vi "禹山溶解氧校准.vi"() -> ()   [LabVIEW 2016, in "斯坦道多参数.lvlib"]
uses:
  <vilib>/Utility/miscctls.llb/LVPointTypeDef.ctl
  <vilib>/Analysis/NI_AALBase.lvlib
  <vilib>/Analysis/NI_AALPro.lvlib
  <vilib>/Utility/config.llb/NI_LVConfig.lvlib
panel:
  out "第二点信号值":dbl
  out "第一点信号值":dbl
  out "通讯状态":string
  in  "盐度自动获取":bool
  in  "大气压补偿":dbl format="%#.2f"
  in  "盐度补偿":dbl format="%#.2f"
  out "DO %":dbl caption="饱和度值" format="%#.2f"
  out "第二点校准值":dbl
  out "第一点校准值":dbl
  out "最小值":sgl format="%.2g"
  out "最大值":sgl format="%.2g"
  in  "校准停止":bool
  in  "校准模式":u16(ring) items=["两点校准", "单点校准"]
  in  "标液2":dbl
  in  "标液1":dbl
  out "波形图表":dbl(graph) caption="历史曲线"
  out "温度测量值":dbl caption="温度" format="%#.2f"
  out "变异系数":dbl format="%.6g"
  out "standard deviation":dbl caption="标准差" format="%0.2f"
  out "mean":dbl caption="均值" format="%0.2f"
  out "提示":string
  in  "校准启动":bool
  out "DO mg/L":dbl caption="测试值" format="%#.2f"
  out "电极斜率":dbl format="%#.6f"
  out "电极零点":dbl format="%#.6f"
  # "溶解氧电极设定"
  # "℃"
  # "%"
  # "mg/L"
  # "kPa"
  # "请选择校准模式:"
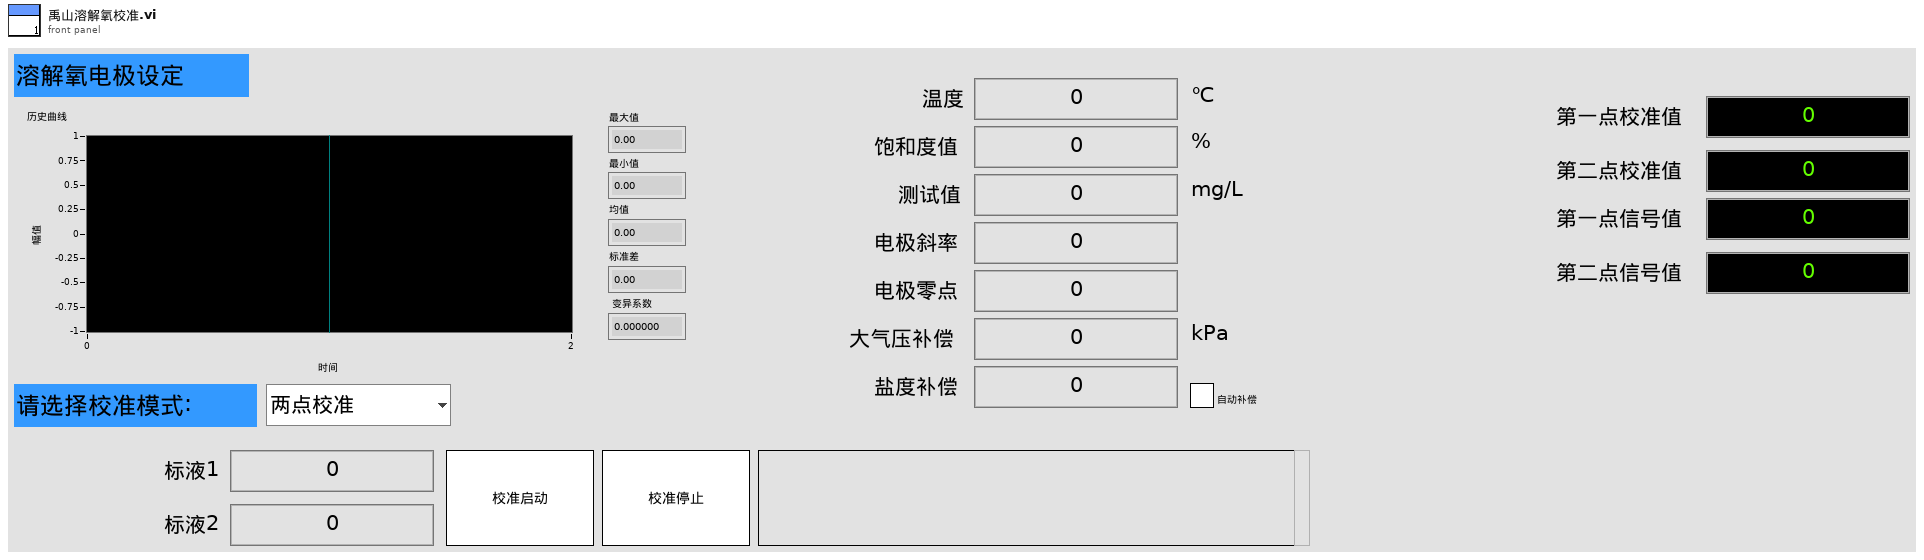
[diagram p1: front panel]
types:
  T1 = typedef "LVPointTypeDef.ctl" = cluster{"Horizontal":i16, "Vertical":i16}
  T2 = typedef "NI_LVConfig.lvlib/Config Data RefNum.ctl" = refnum<k1>
  T3 = enum8{"Enabled", "Disabled", "Disabled and Grayed Out"}
  T4 = cluster{"ph":bool, "DO":bool, "Cond":bool, "Turb":bool, "叶绿素a":bool, "藻密度":bool, "ORP":bool}
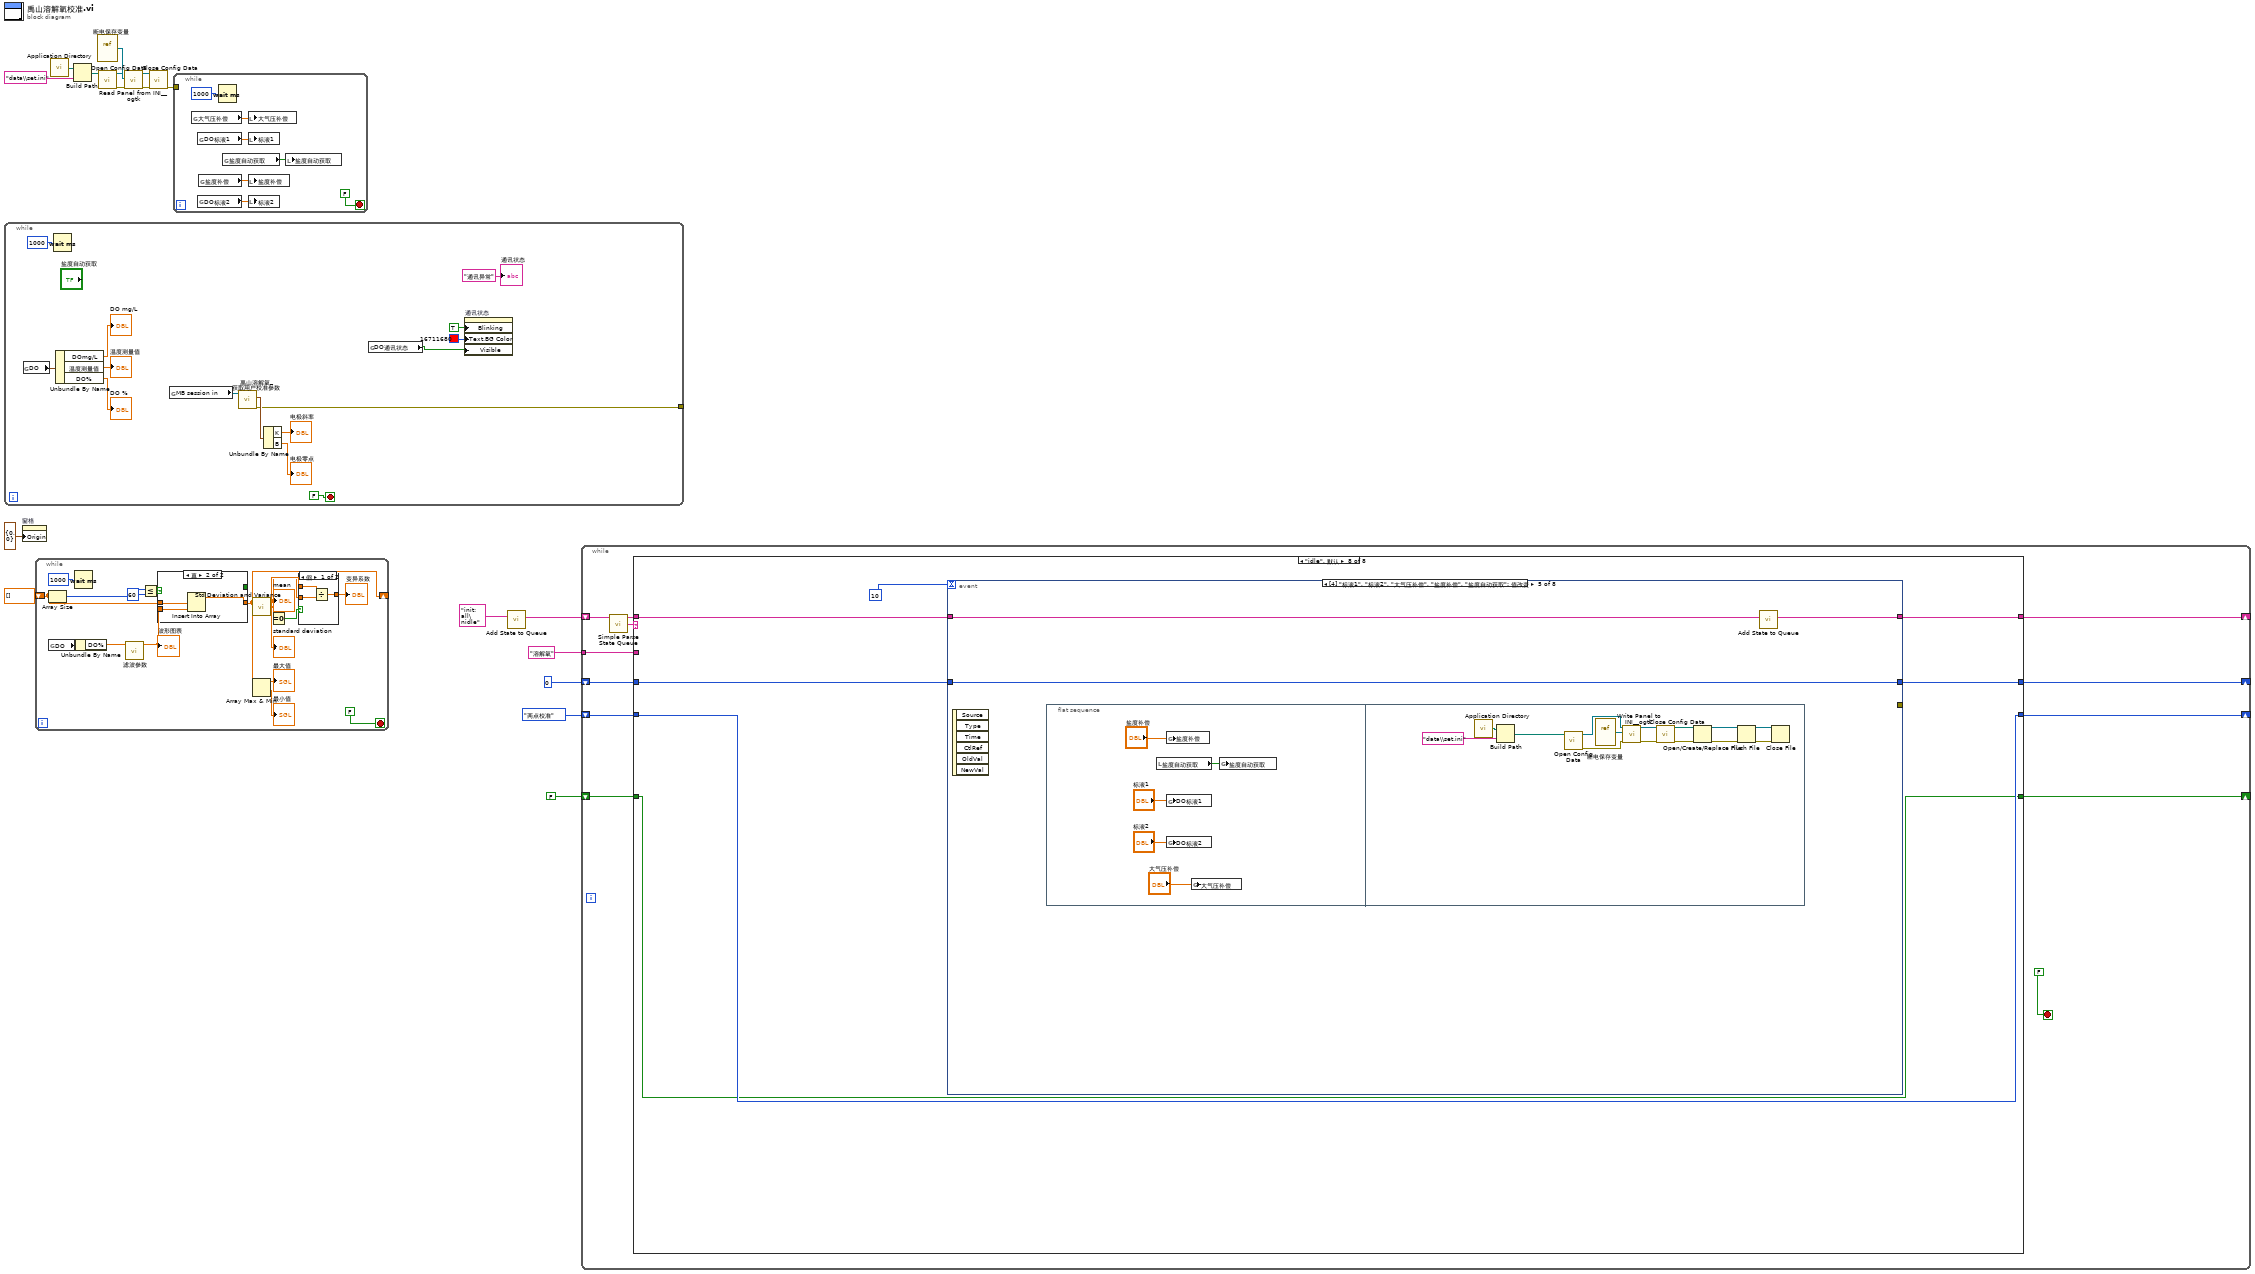
[diagram p0: block diagram]
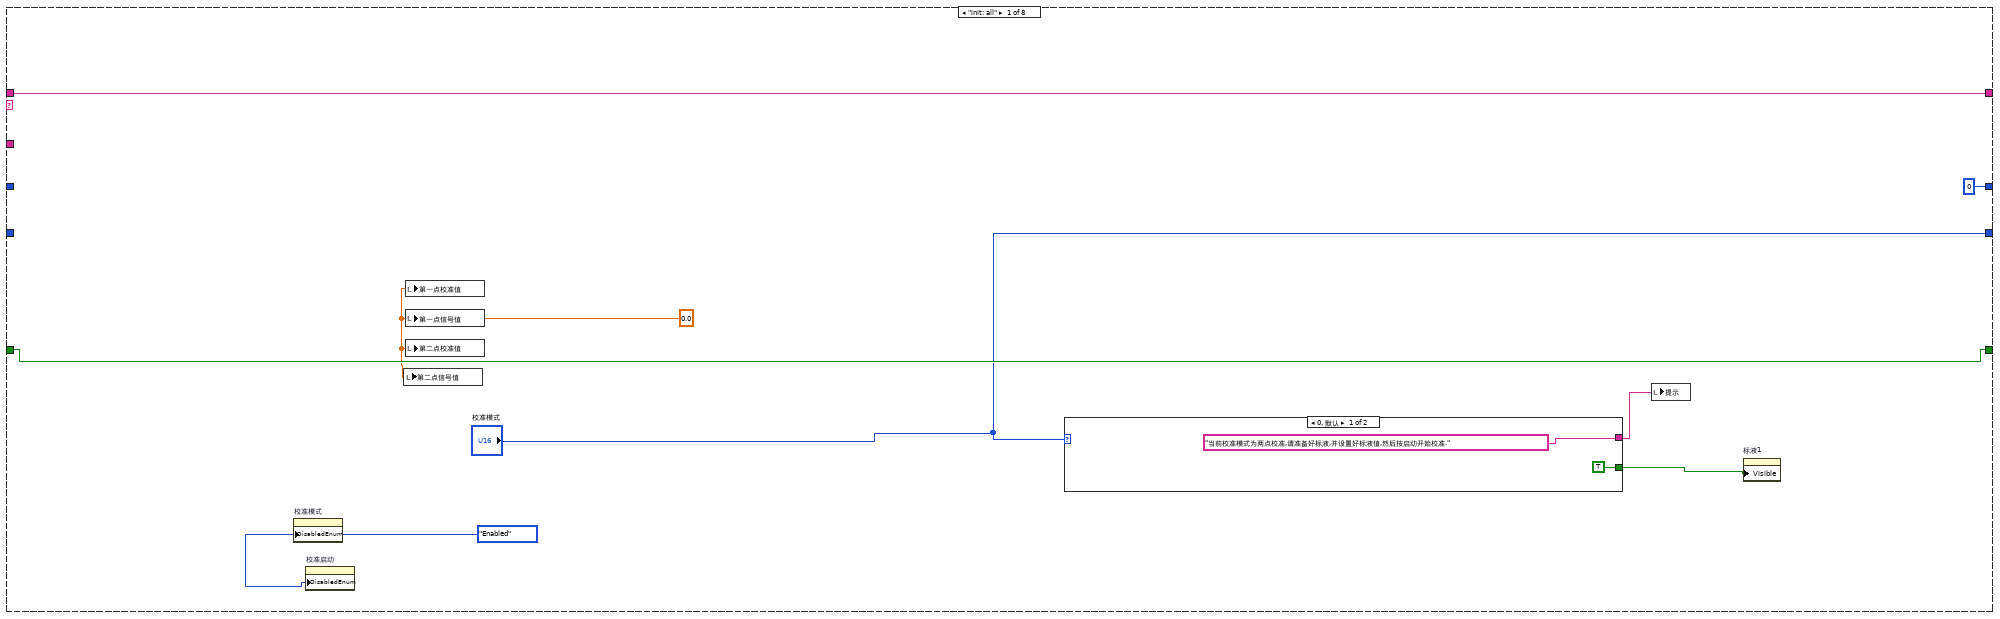
[diagram p2: hidden frame]
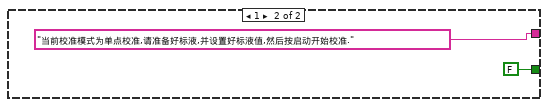
[diagram p3: hidden frame]
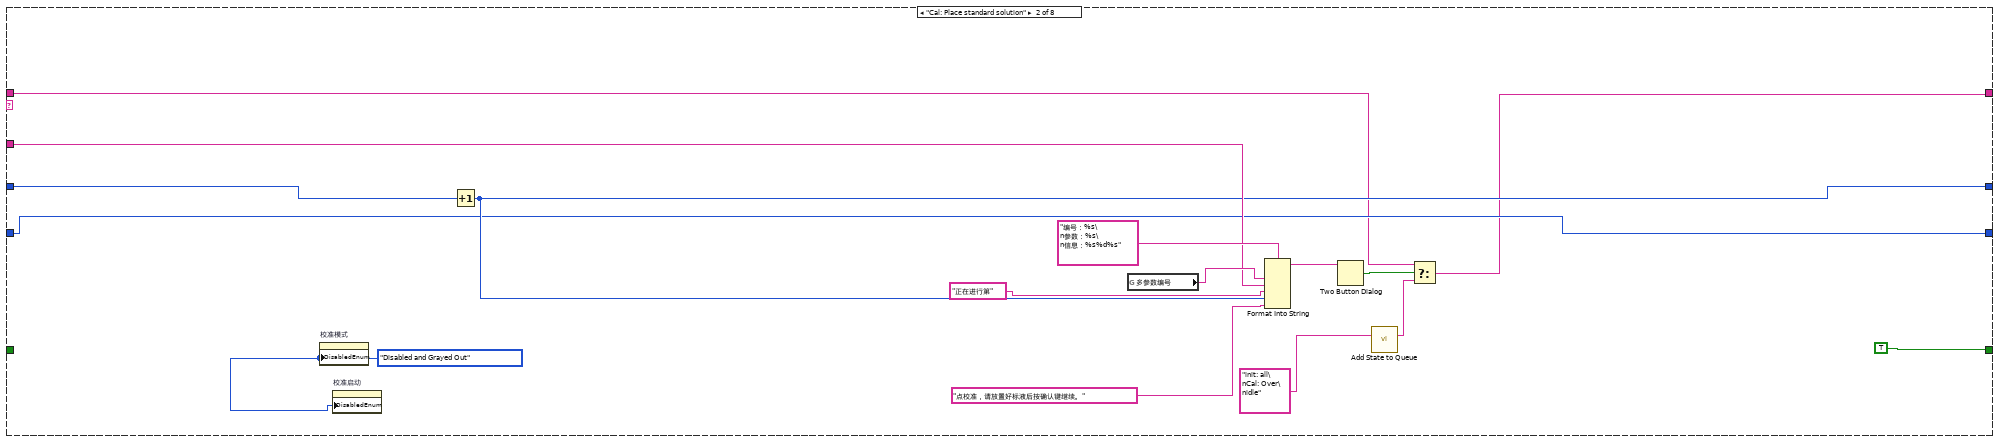
[diagram p4: hidden frame]
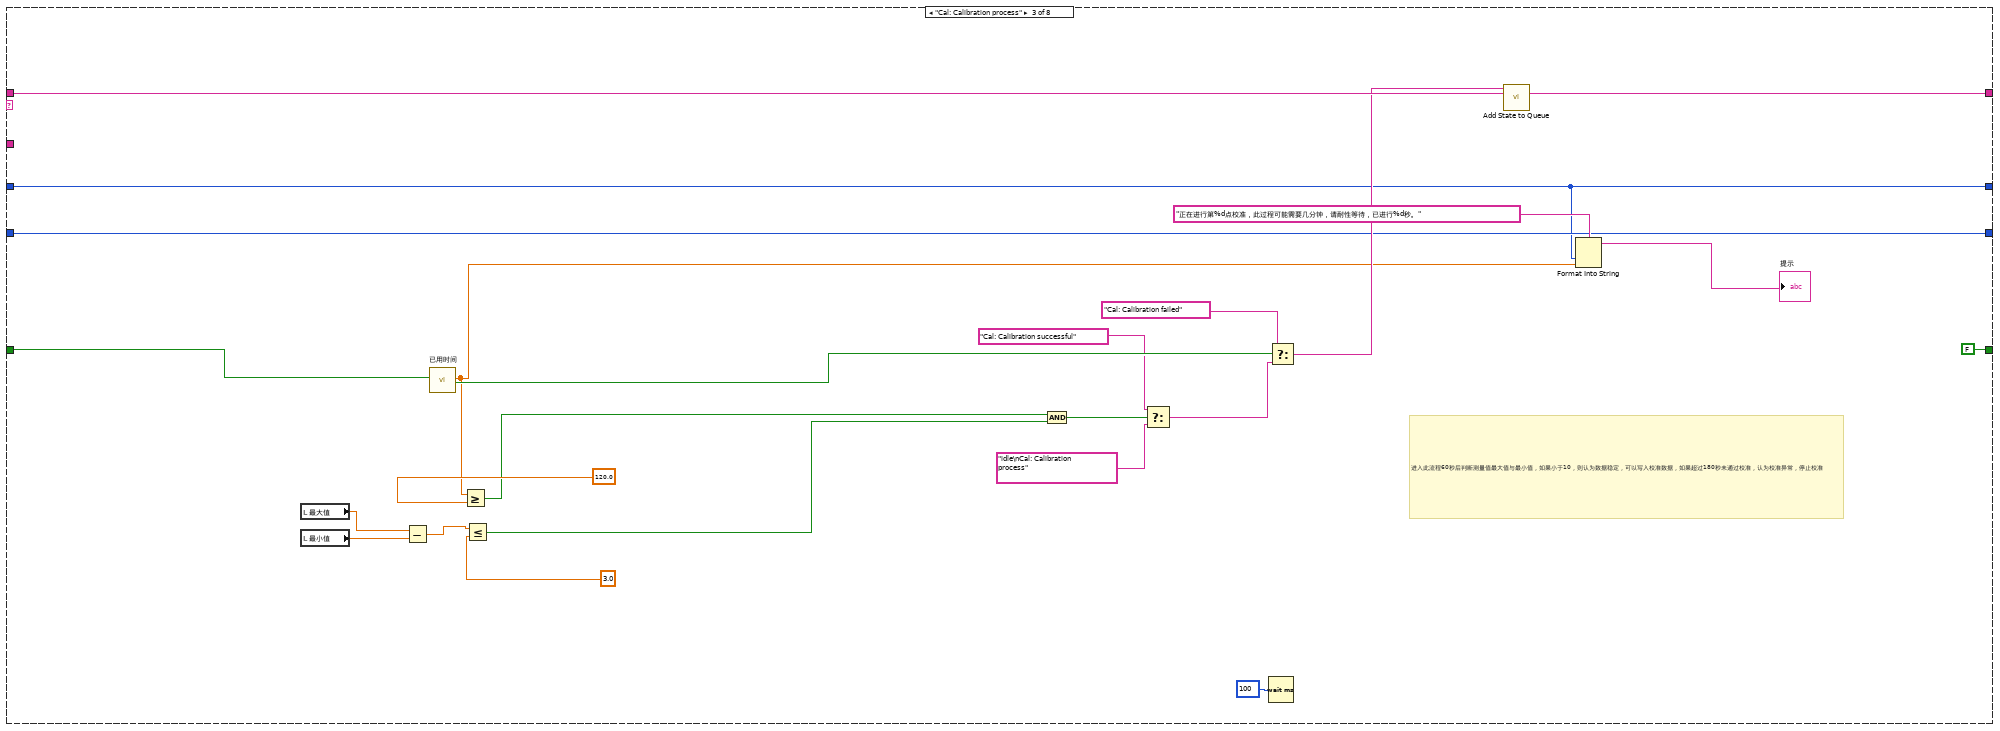
[diagram p5: hidden frame]
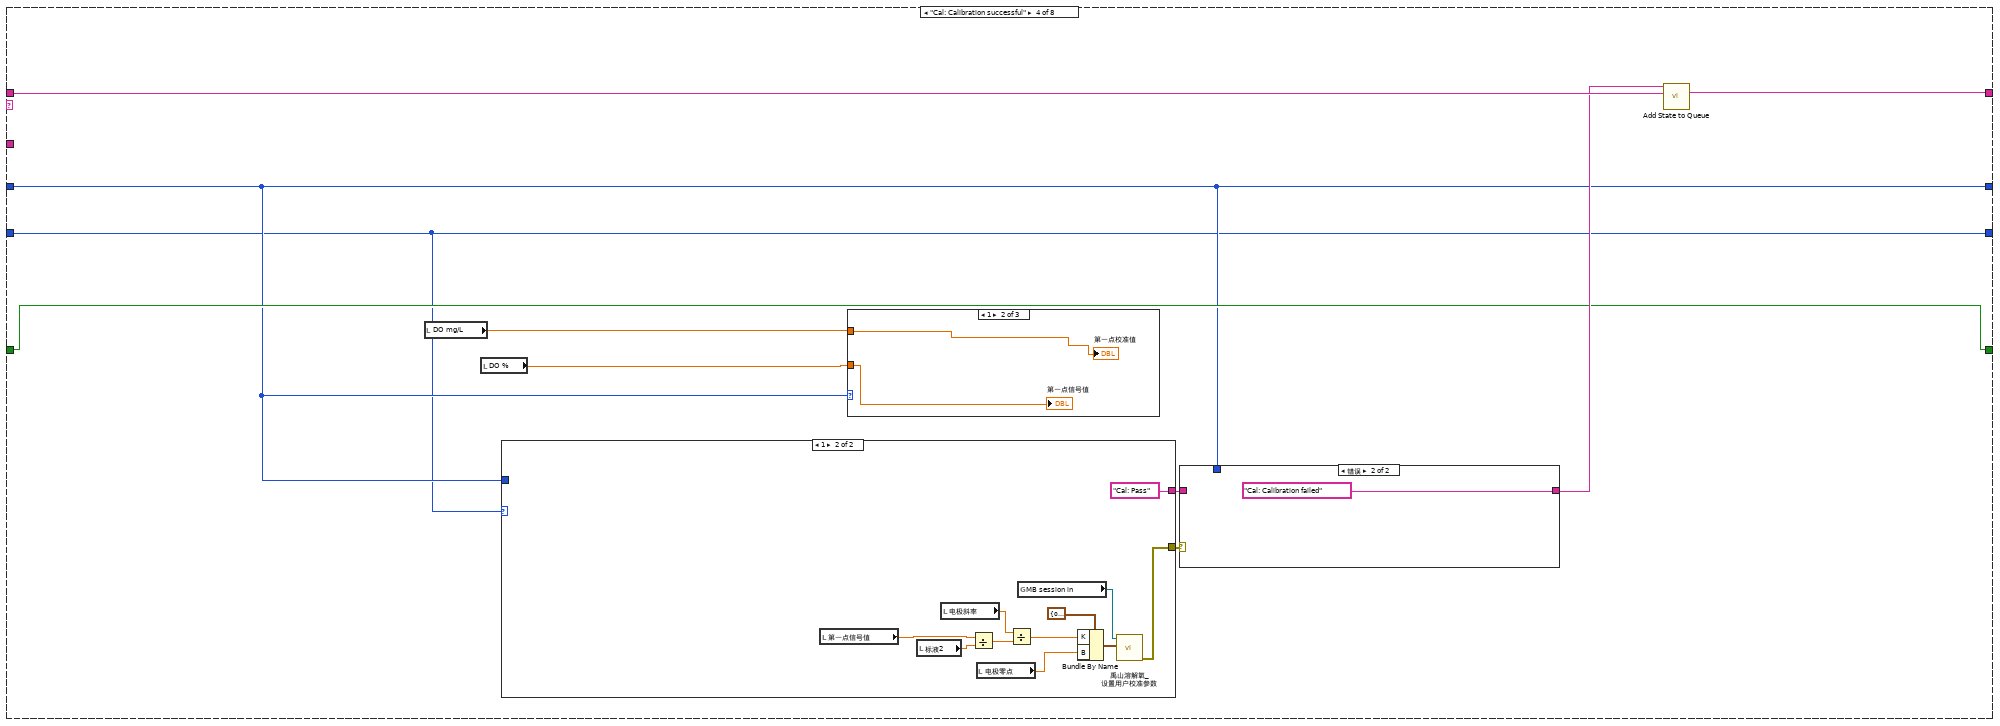
[diagram p6: hidden frame]
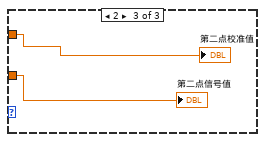
[diagram p8: hidden frame]
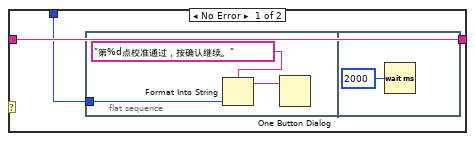
[diagram p9: hidden frame]
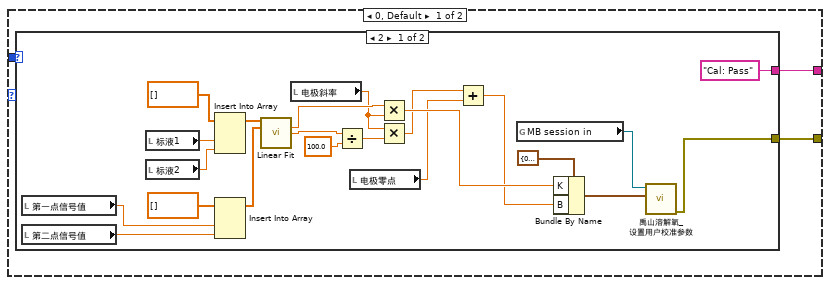
[diagram p10: hidden frame]
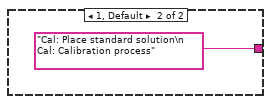
[diagram p11: hidden frame]
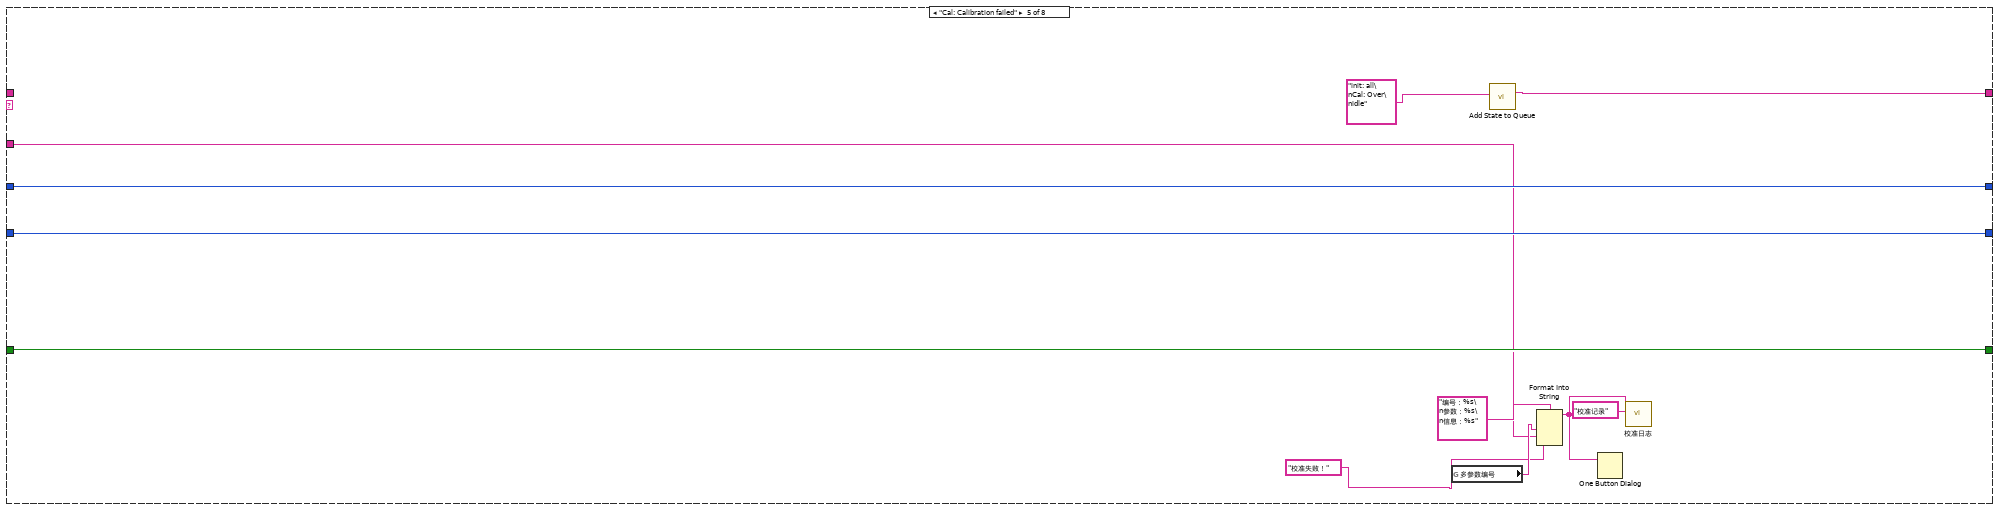
[diagram p12: hidden frame]
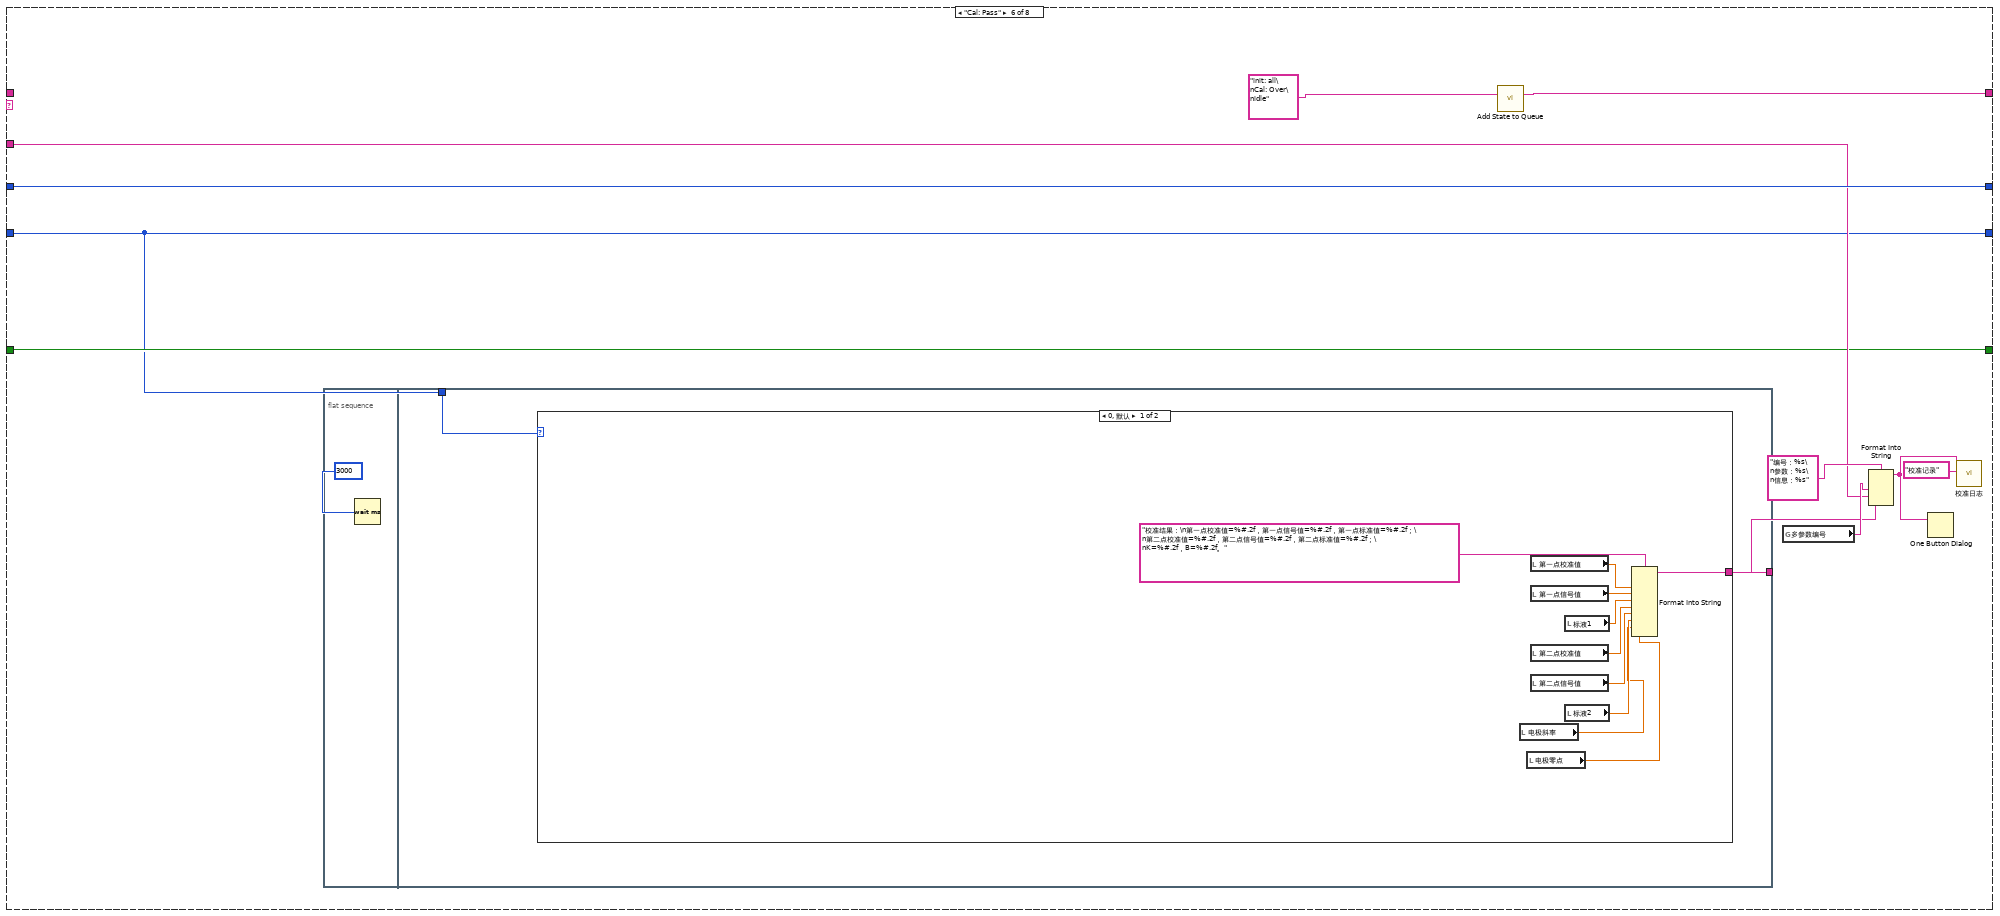
[diagram p13: hidden frame]
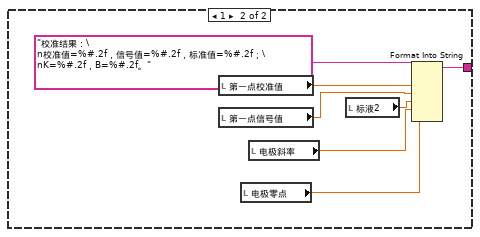
[diagram p14: hidden frame]
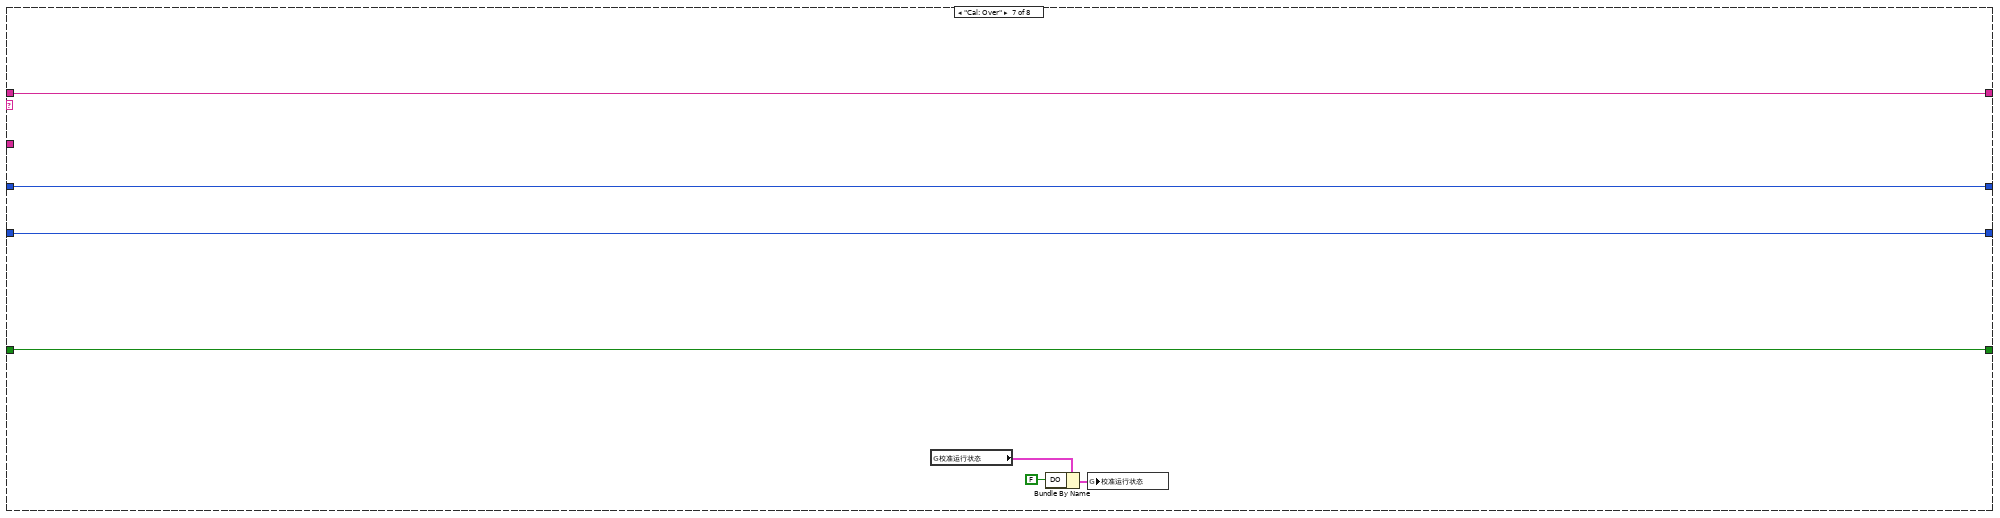
[diagram p15: hidden frame]
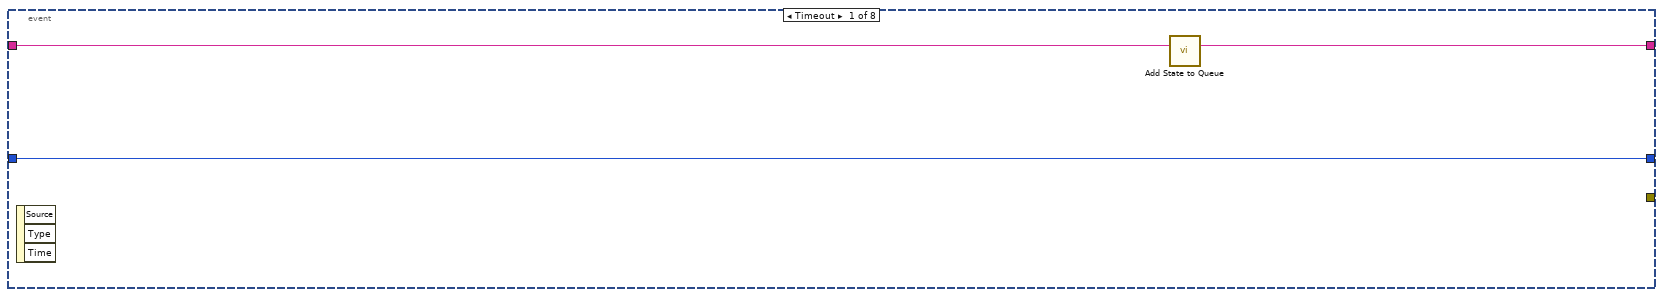
[diagram p16: hidden frame]
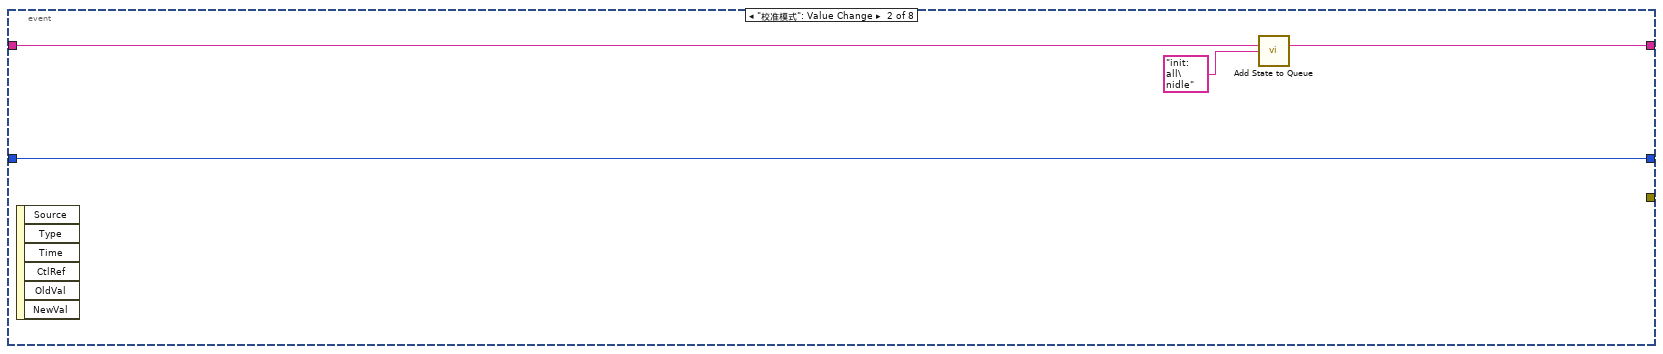
[diagram p17: hidden frame]
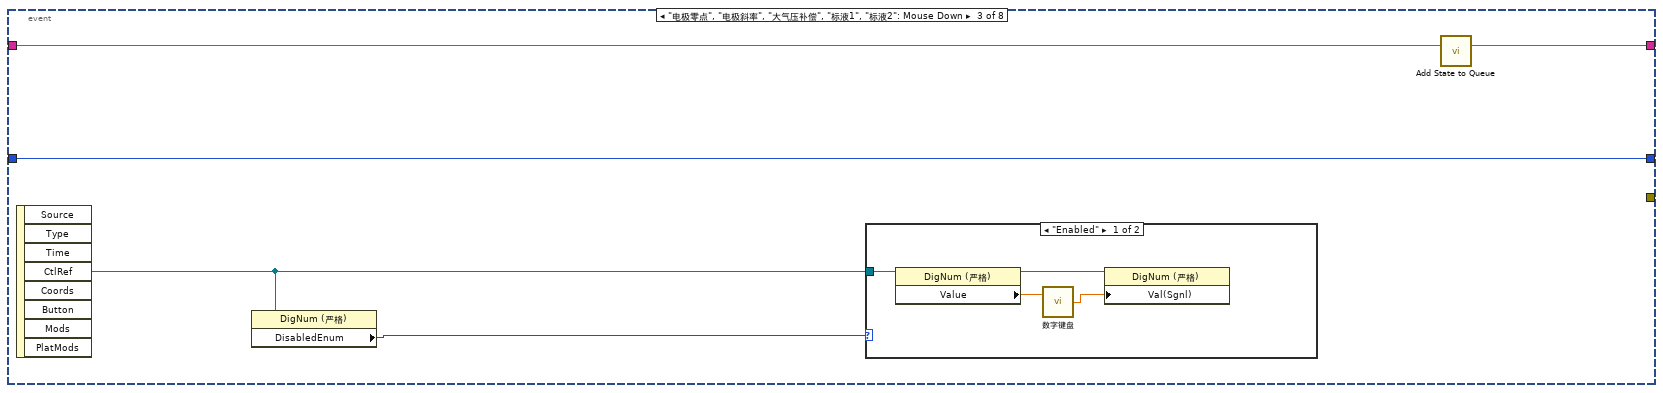
[diagram p18: hidden frame]
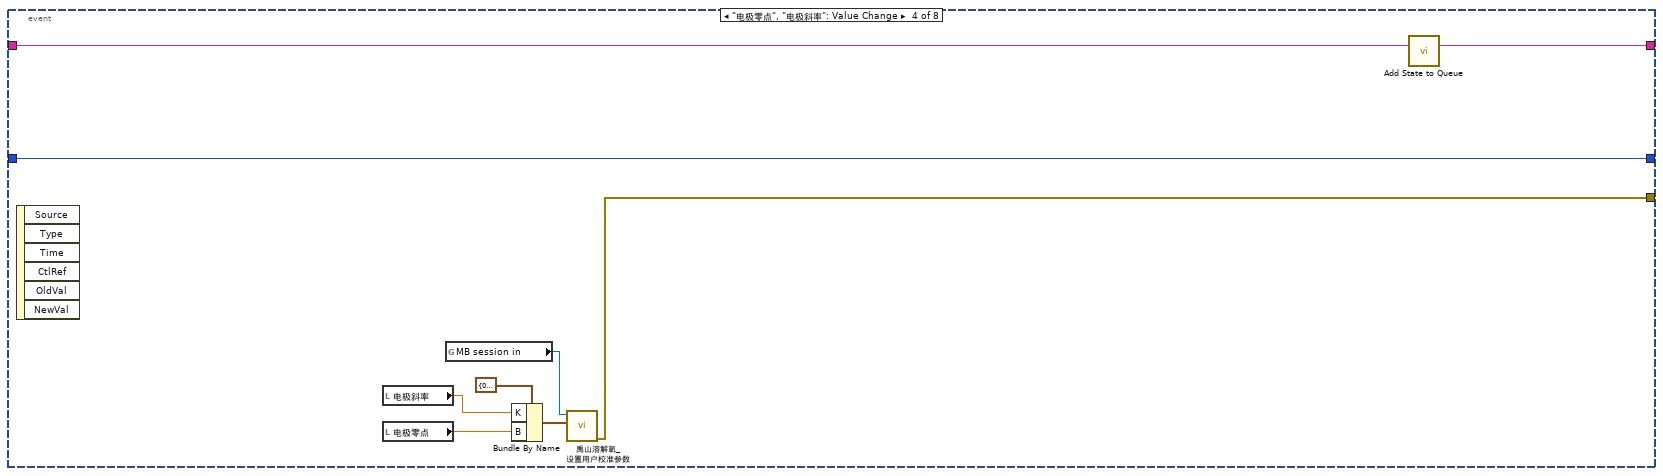
[diagram p20: hidden frame]
diagram:
  n1 = while {
    tunnel: [w27] -> _
    stop <- FALSE stop-if-true
    n2 = global read "禹山过程全局变量.vi" "DO"() -> (w24:cluster{"温度测量值":sgl, "DO%":sgl, "DOmg/L":sgl})
    n3 = Wait (ms)(milliseconds to wait=u32 1000 ("等待时间（毫秒）")) -> ()  [unwired: 1 out]
    n4 = Unbundle By Name(w24) -> ("DOmg/L"=→"DO mg/L":sgl, "温度测量值"=→"温度测量值":sgl, "DO%"=→"DO %":sgl)
    n5 = global read "多参数全局变量.vi" "MB session in"() -> (w23:refnum<class "MB_Master.lvclass">)
    n6 = call "禹山溶解氧_获取用户校准参数.vi"("MB session in"=w23) -> ("error out"=w27:errorcluster, "输出值"=w30:cluster{"K":sgl, "B":sgl})  [unwired: 8 in, 1 out]
    n7 = Unbundle By Name(w30) -> ("K"=→"电极斜率":sgl, "B"=→"电极零点":sgl)
    n8 = global read "多参数全局变量.vi" "DO通讯状态"() -> (w18:bool)
    n9 = property on="通讯状态" class="Str"("Blinking"=TRUE ("闪烁"), "Text.BG Color"=u32 16711680, "Visible"=w18) -> ()  [unwired: 2 in, 2 out]
    "通讯状态" <- "通讯异常" ("当前串口")
  }
  n10 = property on="窗格" class="Pane"("Origin"=T1 {"Horizontal"=0, "Vertical"=0} ("原点")) -> ()  [unwired: 2 in, 2 out]
  n11 = while {
    shift-right: [w37] -> _
    shift-left: sgl[] [] -> [w44]
    stop <- FALSE stop-if-true
    n12 = Array Size(array=w44) -> (size(s)=w46:i32)
    n13 = global read "禹山过程全局变量.vi" "DO"() -> (w38:cluster{"温度测量值":sgl, "DO%":sgl, "DOmg/L":sgl})
    n14 = Wait (ms)(milliseconds to wait=u32 1000 ("等待时间（毫秒）")) -> ()  [unwired: 1 out]
    n15 = Unbundle By Name(w38) -> ("DO%"=w34:sgl)
    n16 = call "滤波参数.vi"("x"=w34) -> ("mode"=w33:dbl)  [unwired: 10 in]
    "波形图表" <- w33
    n17 = Less Or Equal?(x=w46, y=60) -> (x <= y?=w45:bool)
    n18 = case shown="真" w45 {
      tunnel: w44 -> [w57 w60]
      tunnel: w33 -> [w55 w59]
      tunnel: [w53 w58] -> w37
      tunnel: [TRUE _] -> _
      frame False {
        n19 = Replace Array Subset(array=w57, new element=w55) -> (w56:sgl[])  [unwired: 1 in]
        n20 = Rotate 1D Array(1:w56, 2:-1 ("n")) -> (0:w53:sgl[])
      }
      frame True {
        n21 = Insert Into Array(array=w60, new element=w59) -> (w58:sgl[])  [unwired: 1 in]
      }
    }
    n22 = call <vilib>:"Std Deviation and Variance.vi"("X"=w37) -> ("mean"=w39:dbl, "standard deviation"=w40:dbl)  [unwired: 1 in, 1 out]
    "standard deviation" <- w40
    "mean" <- w39
    n23 = Array Max & Min(array=w37) -> (max value=→"最大值":sgl, min value=→"最小值":sgl)  [unwired: 2 out]
    n24 = Equal To 0?(x=w39) -> (x = 0?=w43:bool)
    n25 = case shown="假" w43 {
      tunnel: w40 -> [w51 _]
      tunnel: [w50 _] -> w42
      tunnel: w39 -> [w49 _]
      frame False {
        n26 = Divide(x=w51, y=w49) -> (x/y=w50:dbl)
      }
      frame True {
      }
    }
    "变异系数" <- w42
  }
  n27 = call <vilib>:"Application Directory.vi"() -> ("Application Directory"=w12:path)
  n28 = Build Path(base path=w12, name or relative path="data\\set.ini" ("名称或相对路径")) -> (appended path=w13:path)
  n29 = vi-ref "断电保存变量.vi"() -> (w15:refnum<vi>)
  n30 = call <vilib>:"Open Config Data.vi"("configuration file path"=w13) -> ("error out"=w9:errorcluster, "refnum"=w8:T2)  [unwired: 8 in, 1 out]
  n31 = call <userlib>:"Read Panel from INI__ogtk.vi"("error in (no error)"=w9, "VI ref"=w15, "refnum"=w8) -> ("error out"=w11:errorcluster, "refnum out"=w10:T2)  [unwired: 7 in]
  n32 = call <vilib>:"Close Config Data.vi"("error in (no error)"=w11, "refnum"=w10) -> ("error out"=w7:errorcluster)  [unwired: 8 in, 1 out]
  n33 = while {
    tunnel: w7 -> [_]
    stop <- FALSE stop-if-true
    n34 = global read "断电保存变量.vi" "大气压补偿"() -> (w63:dbl)
    n35 = global read "断电保存变量.vi" "DO标液1"() -> (w65:dbl)
    n36 = global read "断电保存变量.vi" "DO标液2"() -> (w64:dbl)
    n37 = global read "断电保存变量.vi" "盐度补偿"() -> (w61:dbl)
    n38 = Wait (ms)(milliseconds to wait=u32 1000 ("等待时间（毫秒）")) -> ()  [unwired: 1 out]
    n39 = global read "断电保存变量.vi" "盐度自动获取"() -> (w62:bool)
    n40 = local write "大气压补偿"(w63) -> ()
    n41 = local write "标液1"(w65) -> ()
    n42 = local write "盐度补偿"(w61) -> ()
    n43 = local write "标液2"(w64) -> ()
    n44 = local write "盐度自动获取"(w62) -> ()
  }
  n45 = call "Add State to Queue.vi"("State(s) In (\"\")"="init: all\nidle" ("State(s) In (\"\")")) -> ("States Out"=w5:string)  [unwired: 14 in]
  n46 = while {
    shift-right: [w75] -> _
    shift-left: w5 -> [w79]
    shift-right: [w72] -> _
    shift-left: 0 -> [w74]
    tunnel: "溶解氧" ("State(s) In (\"\")") -> [w73]
    shift-right: [w70] -> _
    shift-left: enum16{"两点校准", "单点校准"}."两点校准" ("校准模式") -> [w71]
    shift-right: [w68] -> _
    shift-left: FALSE -> [w69]
    stop <- FALSE stop-if-true
    n47 = call "Simple Parse State Queue.vi"("State Queue"=w79) -> ("Remain States"=w76:string, "Next State"=w77:string)  [unwired: 13 in]
    n48 = case shown="\"idle\", 默认" w77 {
      tunnel: w76 -> [w87 w95 w126 w139 _ _ w238 w245]
      tunnel: [w87 w94 w125 w138 w197 w202 w238 w244] -> w75
      tunnel: w74 -> [_ w103 w110 w133 w200 w211 w237 w242]
      tunnel: w73 -> [_ w104 _ _ w191 w207 _ _]
      tunnel: [0 w101 w110 w133 w200 w211 w237 w243] -> w72
      tunnel: w71 -> [_ w100 w111 w132 w199 w203 w236 w241]
      tunnel: ["校准模式" w100 w111 w132 w199 w203 w236 w241] -> w70
      tunnel: w69 -> [w84 _ w113 w134 w198 w206 w235 w239]
      tunnel: [w84 TRUE FALSE w134 w198 w206 w235 w239] -> w68
      frame "init: all" {
        w82 = T3."Enabled" ("禁用")
        w83 = 0.0 ("第一点校准值")
        n49 = property on="校准模式" class="Ring (严格)"("DisabledEnum"=w82) -> ()  [unwired: 2 in, 2 out]
        n50 = property on="校准启动" class="Bool"("DisabledEnum"=w82) -> ()  [unwired: 2 in, 2 out]
        n51 = local write "第二点信号值"(w83) -> ()
        n52 = local write "第一点校准值"(w83) -> ()
        n53 = local write "第一点信号值"(w83) -> ()
        n54 = local write "第二点校准值"(w83) -> ()
        n55 = case shown="0, 默认" "校准模式" {
          tunnel: ["当前校准模式为两点校准,请准备好标液,并设置好标液值,然后按启动开始校准." ("提示") "当前校准模式为单点校准,请准备好标液,并设置好标液值,然后按启动开始校准." ("提示")] -> w86
          tunnel: [TRUE ("可见") FALSE ("可见")] -> w80
          frame 0, Default {
          }
          frame 1 {
          }
        }
        n56 = local write "提示"(w86) -> ()
        n57 = property on="标液1" class="DigNum (严格)"("Visible"=w80) -> ()  [unwired: 2 in, 2 out]
      }
      frame "Cal: Place standard solution" {
        w93 = T3."Disabled and Grayed Out" ("禁用")
        n58 = property on="校准模式" class="Ring (严格)"("DisabledEnum"=w93) -> ()  [unwired: 2 in, 2 out]
        n59 = property on="校准启动" class="Bool"("DisabledEnum"=w93) -> ()  [unwired: 2 in, 2 out]
        n60 = Increment(x=w103) -> (x+1=w101:i32)
        n61 = global read "多参数全局变量.vi" "多参数编号"() -> (w106:string)
        n62 = Format Into String(format string="编号：%s\n参数：%s\n信息：%s%d%s" ("格式字符串"), w106, w104, "正在进行第" ("消息"), w101, "点校准，请放置好标液后按确认键继续。" ("消息")) -> (resulting string=w98:string)  [unwired: 2 in, 1 out]
        n63 = Two Button Dialog(message=w98) -> (T button?=w97:bool)  [unwired: 2 in]
        n64 = call "Add State to Queue.vi"("State(s) In (\"\")"="init: all\nCal: Over\nidle" ("State(s) In (\"\")")) -> ("States Out"=w96:string)  [unwired: 14 in]
        n65 = Select(t=w95, s=w97, f=w96) -> (s? t:f=w94:string)
      }
      frame "Cal: Calibration process" {
        # "进入此流程60秒后判断测量值最大值与最小值，如果小于10，则认为数据稳定，可以写入校准数据，如果超过180秒未通过校准，认为校准异常，停止校准"
        n66 = local read "最大值"() -> (w130:sgl)
        n67 = local read "最小值"() -> (w129:sgl)
        n68 = Subtract(x=w130, y=w129) -> (x-y=w131:sgl)
        n69 = call "已用时间"("Reset"=w113) -> ("Elapsed Time (s)"=w109:dbl, "Time has Elapsed"=w127:bool)  [unwired: 11 in, 6 out]
        n70 = Greater Or Equal?(x=w109, y=120.0) -> (x >= y?=w122:bool)
        n71 = Less Or Equal?(x=w131, y=3.0) -> (x <= y?=w118:bool)
        n72 = And(x=w122, y=w118) -> (x .and. y?=w119:bool)
        n73 = Select(t="Cal: Calibration successful" ("State(s) In (\"\")"), s=w119, f="idle\nCal: Calibration process" ("State(s) In (\"\")")) -> (s? t:f=w117:string)
        n74 = Wait (ms)(milliseconds to wait=u32 100 ("等待时间（毫秒）")) -> ()  [unwired: 1 out]
        n75 = Select(t="Cal: Calibration failed" ("State(s) In (\"\")"), s=w127, f=w117) -> (s? t:f=w116:string)
        n76 = call "Add State to Queue.vi"("State(s) In Front (\"\")"=w116, "State(s) In (\"\")"=w126) -> ("States Out"=w125:string)  [unwired: 13 in]
        n77 = Format Into String(format string="正在进行第%d点校准，此过程可能需要几分钟，请耐性等待，已进行%d秒。" ("格式字符串"), w110, w109) -> (resulting string=→"提示":string)  [unwired: 2 in, 1 out]
      }
      frame "Cal: Calibration successful" {
        n78 = local read "DO mg/L"() -> (w135:dbl)
        n79 = local read "DO %"() -> (w136:dbl)
        n80 = case shown="1" w132 {
          tunnel: [w155 w179] -> w141
          tunnel: [w154 "Cal: Pass" ("State(s) In (\"\")")] -> w140
          tunnel: w133 -> [w153 _]
          frame 0, Default {
            n81 = case shown="2" w153 {
              tunnel: [w156 _] -> w155
              tunnel: ["Cal: Pass" ("State(s) In (\"\")") "Cal: Place standard solution\n Cal: Calibration process" ("State(s) In (\"\")")] -> w154
              frame 2 {
                n82 = local read "第一点信号值"() -> (w175:dbl)
                n83 = local read "第二点信号值"() -> (w174:dbl)
                n84 = local read "标液1"() -> (w172:dbl)
                n85 = local read "标液2"() -> (w171:dbl)
                n86 = Insert Into Array(array=dbl[] [] ("Weight"), new element #1=w172, new element #2=w171) -> (w170:dbl[])  [unwired: 1 in]
                n87 = Insert Into Array(array=dbl[] [] ("Weight"), new element #1=w175, new element #2=w174) -> (w169:dbl[])  [unwired: 1 in]
                n88 = call <vilib>:"Linear Fit.vi"("Y"=w170, "X"=w169) -> ("slope"=w165:dbl, "intercept"=w162:dbl)  [unwired: 9 in, 3 out]
                n89 = local read "电极斜率"() -> (w163:dbl)
                n90 = Divide(x=w162, y=100.0) -> (x/y=w158:dbl)
                n91 = local read "电极零点"() -> (w160:dbl)
                n92 = Multiply(x=w165, y=w163) -> (x*y=w164:dbl)
                n93 = Multiply(x=w163, y=w158) -> (x*y=w161:dbl)
                n94 = Add(x=w161, y=w160) -> (x+y=w159:dbl)
                n95 = global read "多参数全局变量.vi" "MB session in"() -> (w168:refnum<class "MB_Master.lvclass">)
                n96 = Bundle By Name(cluster=cluster{"K":sgl, "B":sgl} {"K"=0.0, "B"=0.0} ("用户校准参数"), "K"=w164, "B"=w159) -> (w167:cluster{"K":sgl, "B":sgl})
                n97 = call "禹山溶解氧_设置用户校准参数.vi"("用户校准参数"=w167, "MB session in"=w168) -> ("error out"=w156:errorcluster)  [unwired: 8 in, 1 out]
              }
              frame 1, Default {
              }
            }
          }
          frame 1 {
            n98 = local read "第一点信号值"() -> (w184:dbl)
            n99 = local read "标液2"() -> (w183:dbl)
            n100 = local read "电极斜率"() -> (w181:dbl)
            n101 = Divide(x=w184, y=w183) -> (x/y=w180:dbl)
            n102 = local read "电极零点"() -> (w185:dbl)
            n103 = Divide(x=w181, y=w180) -> (x/y=w182:dbl)
            n104 = global read "多参数全局变量.vi" "MB session in"() -> (w188:refnum<class "MB_Master.lvclass">)
            n105 = Bundle By Name(cluster=cluster{"K":sgl, "B":sgl} {"K"=0.0, "B"=0.0} ("用户校准参数"), "K"=w182, "B"=w185) -> (w187:cluster{"K":sgl, "B":sgl})
            n106 = call "禹山溶解氧_设置用户校准参数.vi"("用户校准参数"=w187, "MB session in"=w188) -> ("error out"=w179:errorcluster)  [unwired: 8 in, 1 out]
          }
        }
        n107 = case shown="1" w133 {
          tunnel: w136 -> [_ w143 w145]
          tunnel: w135 -> [_ w142 w144]
          frame 0, Default {
          }
          frame 1 {
            "第一点信号值" <- w143
            "第一点校准值" <- w142
          }
          frame 2 {
            "第二点信号值" <- w145
            "第二点校准值" <- w144
          }
        }
        n108 = case shown="错误" w141 {
          tunnel: w140 -> [w147 _]
          tunnel: [w147 "Cal: Calibration failed" ("State(s) In (\"\")")] -> w137
          tunnel: w133 -> [w146 _]
          frame No Error {
            n109 = flat-sequence {
              tunnel: w146 -> [w148]
              frame #0 {
                n110 = Format Into String(format string="第%d点校准通过，按确认继续。" ("格式字符串"), w148) -> (resulting string=w150:string)  [unwired: 2 in, 1 out]
                n111 = One Button Dialog(message=w150) -> ()  [unwired: 1 in, 1 out]
              }
              frame #1 {
                n112 = Wait (ms)(milliseconds to wait=u32 2000 ("等待时间（毫秒）")) -> ()  [unwired: 1 out]
              }
            }
          }
          frame Error {
          }
        }
        n113 = call "Add State to Queue.vi"("State(s) In Front (\"\")"=w137, "State(s) In (\"\")"=w139) -> ("States Out"=w138:string)  [unwired: 13 in]
      }
      frame "Cal: Calibration failed" {
        n114 = global read "多参数全局变量.vi" "多参数编号"() -> (w194:string)
        n115 = call "Add State to Queue.vi"("State(s) In (\"\")"="init: all\nCal: Over\nidle" ("State(s) In (\"\")")) -> ("States Out"=w197:string)  [unwired: 14 in]
        n116 = Format Into String(format string="编号：%s\n参数：%s\n信息：%s" ("格式字符串"), w194, w191, "校准失败！" ("消息")) -> (resulting string=w193:string)  [unwired: 2 in, 1 out]
        n117 = One Button Dialog(message=w193) -> ()  [unwired: 1 in, 1 out]
        n118 = call "校准日志.vi"("table"="校准记录", "日志信息"=w193) -> ()  [unwired: 9 in, 1 out]
      }
      frame "Cal: Pass" {
        n119 = flat-sequence {
          tunnel: [w214] -> w204
          tunnel: w203 -> [w213]
          frame #0 {
            n120 = Wait (ms)(milliseconds to wait=u32 3000 ("等待时间（毫秒）")) -> ()  [unwired: 1 out]
          }
          frame #1 {
            n121 = case shown="0, 默认" w213 {
              tunnel: [w224 w231] -> w214
              frame 0, Default {
                n122 = local read "电极斜率"() -> (w216:dbl)
                n123 = local read "电极零点"() -> (w215:dbl)
                n124 = local read "第一点校准值"() -> (w222:dbl)
                n125 = local read "第一点信号值"() -> (w223:dbl)
                n126 = local read "第二点校准值"() -> (w219:dbl)
                n127 = local read "第二点信号值"() -> (w218:dbl)
                n128 = local read "标液1"() -> (w220:dbl)
                n129 = local read "标液2"() -> (w217:dbl)
                n130 = Format Into String(format string="校准结果：\n第一点校准值=%#.2f，第一点信号值=%#.2f，第一点标准值=%#.2f；\n第二点校准值=%#.2f，第二点信号值=%#.2f，第二点标准值=%#.2f；\nK=%#.2f，B=%#.2f。" ("提示"), w222, w223, w220, w219, w218, w217, w216, w215) -> (resulting string=w224:string)  [unwired: 2 in, 1 out]
              }
              frame 1 {
                n131 = local read "第一点校准值"() -> (w230:dbl)
                n132 = local read "第一点信号值"() -> (w228:dbl)
                n133 = local read "电极零点"() -> (w225:dbl)
                n134 = local read "电极斜率"() -> (w226:dbl)
                n135 = local read "标液2"() -> (w227:dbl)
                n136 = Format Into String(format string="校准结果：\n校准值=%#.2f，信号值=%#.2f，标准值=%#.2f；\nK=%#.2f，B=%#.2f。" ("提示"), w230, w228, w227, w226, w225) -> (resulting string=w231:string)  [unwired: 2 in, 1 out]
              }
            }
          }
        }
        n137 = call "Add State to Queue.vi"("State(s) In (\"\")"="init: all\nCal: Over\nidle" ("State(s) In (\"\")")) -> ("States Out"=w202:string)  [unwired: 14 in]
        n138 = global read "多参数全局变量.vi" "多参数编号"() -> (w208:string)
        n139 = Format Into String(format string="编号：%s\n参数：%s\n信息：%s" ("格式字符串"), w208, w207, w204) -> (resulting string=w205:string)  [unwired: 2 in, 1 out]
        n140 = One Button Dialog(message=w205) -> ()  [unwired: 1 in, 1 out]
        n141 = call "校准日志.vi"("table"="校准记录", "日志信息"=w205) -> ()  [unwired: 9 in, 1 out]
      }
      frame "Cal: Over" {
        n142 = global read "多参数全局变量.vi" "校准运行状态"() -> (w233:T4)
        n143 = Bundle By Name(cluster=w233, "DO"=FALSE) -> (w234:T4)
        n144 = global write "多参数全局变量.vi" "校准运行状态"(w234) -> ()
      }
      frame "idle", Default {
        n145 = event shown="[4] \"标液1\", \"标液2\", \"大气压补偿\", \"盐度补偿\", \"盐度自动获取\": 值改变" {
          selector: _ -> [_ _ _ _ _ _ _ _]
          dyn-events: _ -> [_ _ _ _ _ _ _ _]
          timeout: 10 -> [_ _ _ _ _ _ _ _]
          tunnel: [_ _ _ w263 _ _ _ _] -> _
          tunnel: w245 -> [w248 w252 w255 w262 w271 w293 w308 _]
          tunnel: [w247 w251 w256 w269 w272 w295 w307 w310] -> w244
          tunnel: [w246 w249 w257 w270 w273 w294 w305 w311] -> w243
          tunnel: w242 -> [w246 w249 w257 w270 w273 w294 w305 w311]
          event Timeout {
            n146 = event-data() -> ()  [unwired: 1 in, 3 out]
            n147 = call "Add State to Queue.vi"("State(s) In (\"\")"=w248) -> ("States Out"=w247:string)  [unwired: 14 in]
          }
          event "校准模式": Value Change {
            n148 = event-data() -> ()  [unwired: 1 in, 6 out]
            n149 = call "Add State to Queue.vi"("State(s) In (\"\")"=w252, "State(s) At Back (\"\")"="init: all\nidle" ("State(s) In (\"\")")) -> ("States Out"=w251:string)  [unwired: 13 in]
          }
          event "电极零点", "电极斜率", "大气压补偿", "标液1", "标液2": Mouse Down {
            n150 = event-data() -> ("CtlRef"=w254:refnum<vi>)  [unwired: 1 in, 7 out]
            n151 = property class="DigNum (严格)"(reference=w254) -> ("DisabledEnum"=w253:T3)  [unwired: 1 in, 2 out]
            n152 = case shown="\"Enabled\"" w253 {
              tunnel: w254 -> [w261 _]
              frame "Enabled" {
                n153 = property class="DigNum (严格)"(reference=w261) -> (reference out=w258:refnum<vi>, "Value"=w259:dbl)  [unwired: 1 in, 1 out]
                n154 = call "数字键盘.vi"("OldNumber"=w259) -> ("NewNumber"=w260:dbl)  [unwired: 1 in]
                n155 = property class="DigNum (严格)"(reference=w258, "Val(Sgnl)"=w260) -> ()  [unwired: 1 in, 2 out]
              }
              frame "Disabled", Default {
              }
            }
            n156 = call "Add State to Queue.vi"("State(s) In (\"\")"=w255) -> ("States Out"=w256:string)  [unwired: 14 in]
          }
          event "电极零点", "电极斜率": Value Change {
            n157 = event-data() -> ()  [unwired: 1 in, 6 out]
            n158 = local read "电极斜率"() -> (w266:dbl)
            n159 = local read "电极零点"() -> (w265:dbl)
            n160 = global read "多参数全局变量.vi" "MB session in"() -> (w264:refnum<class "MB_Master.lvclass">)
            n161 = Bundle By Name(cluster=cluster{"K":sgl, "B":sgl} {"K"=0.0, "B"=0.0} ("用户校准参数"), "K"=w266, "B"=w265) -> (w267:cluster{"K":sgl, "B":sgl})
            n162 = call "禹山溶解氧_设置用户校准参数.vi"("用户校准参数"=w267, "MB session in"=w264) -> ("error out"=w263:errorcluster)  [unwired: 8 in, 1 out]
            n163 = call "Add State to Queue.vi"("State(s) In (\"\")"=w262) -> ("States Out"=w269:string)  [unwired: 14 in]
          }
          event "标液1", "标液2", "大气压补偿", "盐度补偿", "盐度自动获取": Value Change {
            n164 = event-data() -> ()  [unwired: 1 in, 6 out]
            n165 = flat-sequence {
              frame #0 {
                n166 = local read "盐度自动获取"() -> (w274:bool)
                n167 = global write "断电保存变量.vi" "盐度补偿"("盐度补偿") -> ()
                n168 = global write "断电保存变量.vi" "DO标液1"("标液1") -> ()
                n169 = global write "断电保存变量.vi" "DO标液2"("标液2") -> ()
                n170 = global write "断电保存变量.vi" "大气压补偿"("大气压补偿") -> ()
                n171 = global write "断电保存变量.vi" "盐度自动获取"(w274) -> ()
              }
              frame #1 {
                n172 = call <vilib>:"Application Directory.vi"() -> ("Application Directory"=w288:path)
                n173 = Build Path(base path=w288, name or relative path="data\\set.ini" ("名称或相对路径")) -> (appended path=w287:path)
                n174 = call <vilib>:"Open Config Data.vi"("configuration file path"=w287) -> ("error out"=w291:errorcluster, "refnum"=w292:T2)  [unwired: 8 in, 1 out]
                n175 = vi-ref "断电保存变量.vi"() -> (w285:refnum<vi>)
                n176 = call <userlib>:"Write Panel to INI__ogtk.vi"("error in (no error)"=w291, "VI ref"=w285, "refnum"=w292) -> ("error out"=w289:errorcluster, "refnum out"=w290:T2)  [unwired: 7 in]
                n177 = call <vilib>:"Close Config Data.vi"("error in (no error)"=w289, "refnum"=w290) -> ("error out"=w281:errorcluster, "file path"=w282:path)  [unwired: 8 in]
                n178 = Open/Create/Replace File(file path (use dialog)=w282, error in=w281) -> (refnum out=w283:refnum<file>, error out=w284:errorcluster)  [unwired: 4 in, 1 out]
                n179 = Flush File(refnum=w283, error in=w284) -> (refnum out=w279:refnum<file>, error out=w280:errorcluster)
                n180 = Close File(refnum=w279, error in=w280) -> ()  [unwired: 2 out]
              }
            }
            n181 = call "Add State to Queue.vi"("State(s) In (\"\")"=w271) -> ("States Out"=w272:string)  [unwired: 14 in]
          }
          event "盐度补偿": Mouse Down {
            n182 = event-data() -> ("CtlRef"=w296:refnum<vi>)  [unwired: 1 in, 7 out]
            n183 = local read "盐度自动获取"() -> (w297:bool)
            n184 = case shown="假" w297 {
              tunnel: w296 -> [w298 _]
              frame False {
                n185 = property class="DigNum (严格)"(reference=w298) -> (reference out=w299:refnum<vi>, "Value"=w300:dbl)  [unwired: 1 in, 1 out]
                n186 = call "数字键盘.vi"("OldNumber"=w300) -> ("NewNumber"=w301:dbl)  [unwired: 1 in]
                n187 = property class="DigNum (严格)"(reference=w299, "Val(Sgnl)"=w301) -> ()  [unwired: 1 in, 2 out]
              }
              frame True {
              }
            }
            n188 = call "Add State to Queue.vi"("State(s) In (\"\")"=w293) -> ("States Out"=w295:string)  [unwired: 14 in]
          }
          event "校准启动": Value Change {
            n189 = event-data() -> ()  [unwired: 1 in, 6 out]
            n190 = global read "多参数全局变量.vi" "校准运行状态"() -> (w303:T4)
            n191 = Bundle By Name(cluster=w303, "DO"=TRUE) -> (w304:T4)
            n192 = call "Add State to Queue.vi"("State(s) In (\"\")"=w308, "State(s) At Back (\"\")"="init: all\nCal: Place standard solution\n Cal: Calibration process\nidle" ("State(s) In (\"\")")) -> ("States Out"=w307:string)  [unwired: 13 in]
            n193 = global write "多参数全局变量.vi" "校准运行状态"(w304) -> ()
          }
          event "校准停止": Value Change {
            n194 = event-data() -> ()  [unwired: 1 in, 6 out]
            n195 = call "Add State to Queue.vi"("State(s) In (\"\")"="init: all\nCal: Over\nidle" ("State(s) In (\"\")")) -> ("States Out"=w310:string)  [unwired: 14 in]
          }
        }
      }
    }
  }
